vi "Error Handler.vi"(8 "error in (no error)":errorcluster, 9 "return code":i32, 10 "standard error":string) -> (0 "error out":errorcluster)   [LabVIEW 2019, in "Git.lvclass"]
uses:
  Git.lvclass
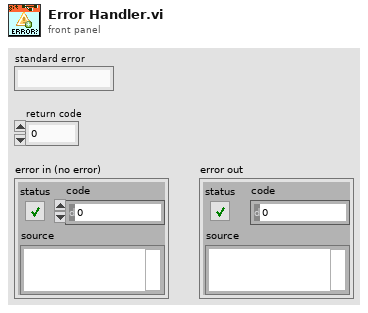
[diagram p1: front panel]
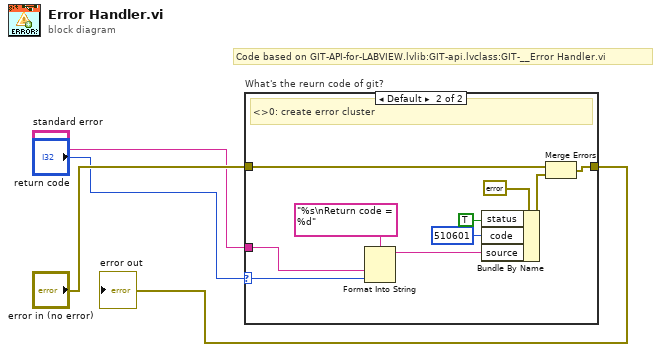
[diagram p0: block diagram]
diagram:
  # "Code based on GIT-API-for-LABVIEW.lvlib:GIT-api.lvclass:GIT-__Error Handler.vi"
  n1 = case "What's the reurn code of git?" shown="Default" "return code" {
    selector: "return code" -> [_ w10]
    tunnel: "standard error" -> [_ w11]
    tunnel: "error in (no error)" -> [w5 w9]
    tunnel: [w5 w6] -> w4
    frame 0 {
      # "0: all well"
    }
    frame Default {
      # "<>0: create error cluster"
      n2 = Format Into String(format string="%s\nReturn code = %d", w11, w10) -> (resulting string=w14:string)  [unwired: 2 in, 1 out]
      n3 = Bundle By Name(cluster=errorcluster {"status"=FALSE, "code"=0, "source"=""} ("error IO"), "status"=TRUE, "code"=510601, "source"=w14) -> (w7:errorcluster)
      n4 = Merge Errors(w9, w7) -> (w6:errorcluster)
    }
  }
  "error out" <- w4
